vi "温度校准写入.vi"(8 "Error in":errorcluster caption="Error in (no error)", 9 "B 2":dbl caption="温度校准值B:", 10 "K 2":dbl caption="温度校准值K:", 11 "站号":u16(ring)=10 items=["氨氮"=3, "水温"=9, "pH值"=10, "溶解氧"=11, "电导率"=12, "浊度"=13, "叶绿素a"=14, "藻密度"=15, "蓝绿藻"=16, "氧化还原电位"=17, "溶解氧%"=18, "盐度"=19]) -> (0 "error out":errorcluster)   [LabVIEW 2016, in "斯坦道原位多参数.lvlib"]
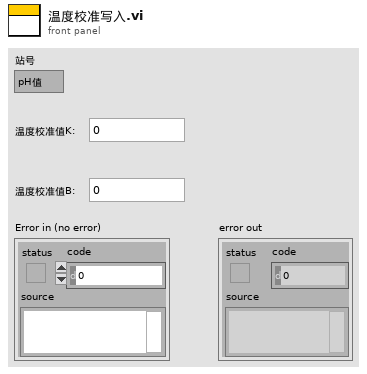
[diagram p1: front panel]
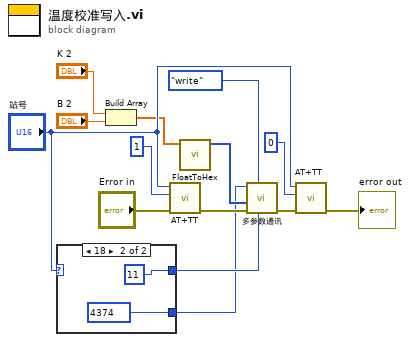
[diagram p0: block diagram]
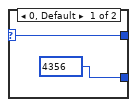
[diagram p2: hidden frame]
diagram:
  n1 = case shown="18" "站号" {
    selector: "站号" -> [w16 _]
    tunnel: [w16 u16 11 ("站号")] -> w6
    tunnel: [u16 4356 ("starting address") u16 4374 ("starting address")] -> w1
    frame 0, Default {
    }
    frame 18 {
    }
  }
  n2 = Build Array("K 2", "B 2") -> (w5:dbl[])
  n3 = call "AT+TT.vi"("错误输入（无错误）"="Error in", "Count"=1, "站号"="站号") -> ("错误输出"=w4:errorcluster)  [unwired: 7 in, 1 out]
  n4 = call "FloatToHex.vi"("浮点数"=w5) -> ("DCBA整形输出"=w2:u16[])  [unwired: 10 in]
  n5 = call "多参数通讯.vi"("Slave ID"=w6, "STEP"=enum16{"open", "read", "write", "close"}."write", "Error in"=w4, "values"=w2, "starting address"=w1) -> ("error out"=w13:errorcluster)  [unwired: 4 in, 2 out]
  n6 = call "AT+TT.vi"("错误输入（无错误）"=w13, "Count"=0, "站号"="站号") -> ("错误输出"=→"error out":errorcluster)  [unwired: 7 in, 1 out]
